vi "Find VI.vi"(8 "error in (no error)":errorcluster, 10 "name":string, 11 "Library in":refnum<vi>) -> (0 "error out":errorcluster, 3 "VI Reference":refnum<vi>)   [LabVIEW 2024, in "UI.lvlib"]
uses:
  UI.lvlib
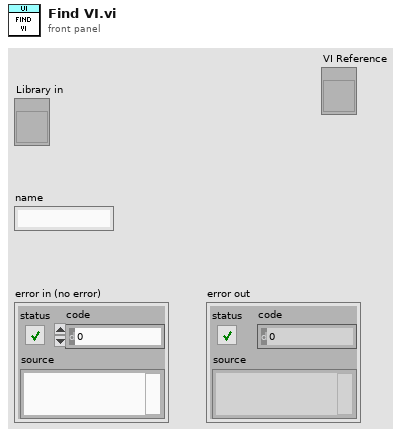
[diagram p1: front panel]
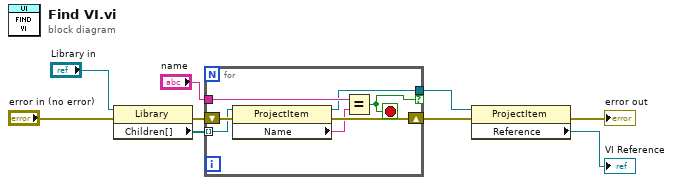
[diagram p0: block diagram]
diagram:
  n1 = property class="Library"(reference="Library in", error in="error in (no error)") -> (error out=w5:errorcluster, "Children[]"=w8:refnum<vi>[])  [unwired: 1 out]
  n2 = for {
    tunnel: w8 -> [w14] mode=indexing
    shift-right: [w15] -> w7
    shift-left: w5 -> [w16]
    tunnel: "name" -> [w12]
    tunnel: [w11] -> w2 if=w10
    stop <- w10 stop-if-true
    n3 = property class="ProjectItem"(reference=w14, error in=w16) -> (reference out=w11:refnum<vi>, error out=w15:errorcluster, "Name"=w13:string)
    n4 = Equal?(x=w12, y=w13) -> (x = y?=w10:bool)
  }
  n5 = property class="ProjectItem"(reference=w2, error in=w7) -> (error out=→"error out":errorcluster, "Reference"=→"VI Reference":refnum<vi>)  [unwired: 1 out]
